vi "Read EEPROM.vi"() -> ()   [LabVIEW 2011, in "Wiimote.lvlib"]
uses:
  Wiimote.lvlib
  Wiimote Address Space.ctl
panel:
  out "error out":errorcluster
  in  "Address Space":T1 items=["EEPROM Memory"=0, "Control Register"=4]
  in  "index":i32
  out "Size out":i32
  in  "Size in":u16=16
  in  "Offset":u32 format="%06x"
  out "pReportBuffer out":u8[](array[numeric]) format="%02x"
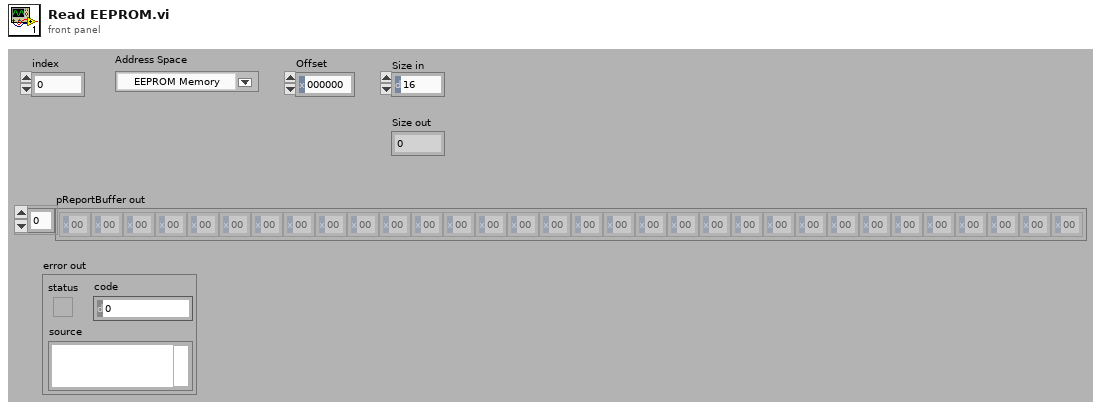
[diagram p1: front panel]
types:
  T1 = typedef "Wiimote.lvlib/Wiimote Address Space.ctl" = u8
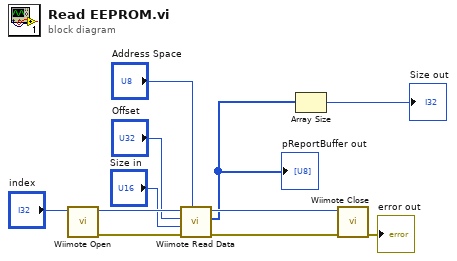
[diagram p0: block diagram]
diagram:
  n1 = call "Wiimote Open.vi"("index"="index") -> ("error out"=w11:errorcluster, "hWiimoteHandle"=w10:u32)  [unwired: 9 in]
  n2 = call "Wiimote Read Data.vi"("Address Space"="Address Space", "error in"=w11, "Size"="Size in", "Offset"="Offset", "hWiimoteHandle in"=w10) -> ("error out"=w6:errorcluster, "pReportBuffer out"=w5:u8[], "hWiimoteHandle out"=w7:u32)  [unwired: 4 in]
  "pReportBuffer out" <- w5
  n3 = Array Size(array=w5) -> (size(s)=→"Size out":i32)
  n4 = call "Wiimote Close.vi"("error in"=w6, "hWiimoteHandle in"=w7) -> ("error out"=→"error out":errorcluster)  [unwired: 9 in]
